vi "INIT sensors.vi"(8 "error in (no error)":errorcluster) -> (0 "error out":errorcluster)   [LabVIEW 2023]
uses:
  Global INIT.vi
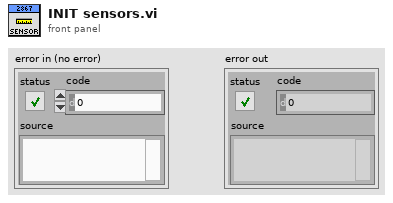
[diagram p1: front panel]
types:
  T1 = typedef "ctrl DIO.ctl" = cluster{"description":string, "Installed?":bool, "DIOChannel":T2, "refnum name":string}
  T2 = typedef "FPGA_DIOChannel.ctl" = enum8{"DIO 0", "DIO 1", "DIO 2", "DIO 3", "DIO 4", "DIO 5", "DIO 6", "DIO 7", "DIO 8", "DIO 9", "DIO MXP 0", "DIO MXP 1", "DIO MXP 2", "DIO MXP 3", "DIO MXP 4", "DIO MXP 5", "DIO MXP 6", "DIO MXP 7", "DIO MXP 8", "DIO MXP 9", "DIO MXP 10", "DIO MXP 11", "DIO MXP 12", "DIO MXP 13", "DIO MXP 14", "DIO MXP 15", "SPI Port CS1", "SPI Port CS2", "SPI Port CS3", "SPI Port MISO", "SPI Port MOSI", "Invalid"}
  T3 = typedef "WPI_DigitalInputDevRef.ctl" = cluster{"DevStatus":errorcluster, "DIO Channel":T2}
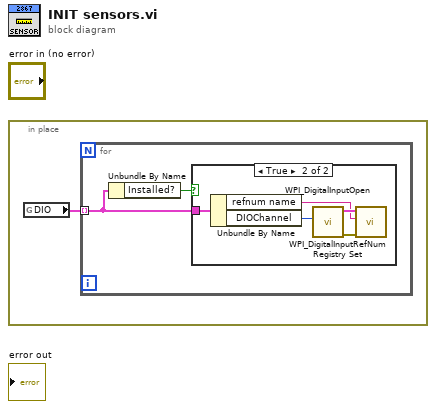
[diagram p0: block diagram]
diagram:
  n1 = in-place {
    n2 = global read "Global INIT.vi" "DIO"() -> (w1:T1[])
    n3 = for {
      tunnel: w1 -> [w2] mode=indexing
      n4 = Unbundle By Name(w2) -> ("Installed?"=w3:bool)
      n5 = case shown="True" w3 {
        tunnel: w2 -> [_ w6]
        frame False {
        }
        frame True {
          n6 = Unbundle By Name(w6) -> ("refnum name"=w4:string, "DIOChannel"=w5:T2)
          n7 = call <vilib>:"WPI_DigitalInputOpen.vi"("DIO Channel"=w5) -> ("error out"=w8:errorcluster, "DigitalInputDevRef"=w7:T3)  [unwired: 9 in]
          n8 = call <vilib>:"WPI_DigitalInputRefNum Registry Set.vi"("error in (no error)"=w8, "refnum name"=w4, "DigitalInputDevRef"=w7) -> ()  [unwired: 7 in, 2 out]
        }
      }
    }
  }
